vi "VCS Set Operation Mode.vi"(8 "error in (no error)":errorcluster, 10 "modes of operations":i8(ring)=1 items=["Profile Position Mode"=1, "Profile Velocity Mode"=3, "Homing Mode"=6, "Interpolated Position Mode"=7, "Position Mode"=-1, "Velocity Mode"=-2, "Current Mode"=-3, "Master Encoder Mode"=-5, "Step Direction Mode"=-6], 11 "axis in":cluster{"keyHandle":u32, "nodeId":u16}={"keyHandle"=0, "nodeId"=1}) -> (0 "error out":errorcluster, 3 "axis out":cluster{"keyHandle":u32, "nodeId":u16}={"keyHandle"=0, "nodeId"=1})   [LabVIEW 2018]
doc: "<B>VCS Set Operation Mode</B> sets the operation mode."
uses:
  Resources/EposCmd.dll
  Resources/EposCmd64.dll
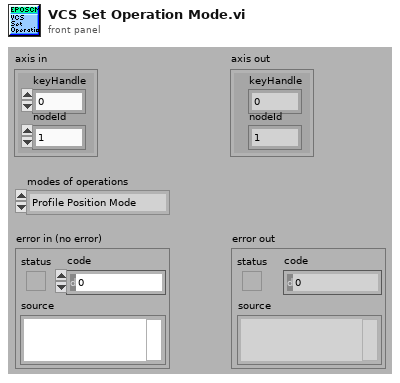
[diagram p1: front panel]
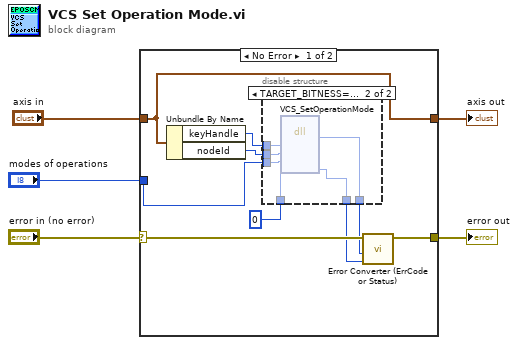
[diagram p0: block diagram]
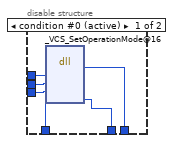
[diagram p2: hidden frame]
diagram:
  n1 = case shown="No Error" "error in (no error)" {
    selector: "error in (no error)" -> [w14 w28]
    tunnel: [w13 w28] -> w4
    tunnel: "modes of operations" -> [w11 _]
    tunnel: "axis in" -> [w8 w27]
    tunnel: [w8 w27] -> w1
    frame No Error {
      n2 = Unbundle By Name(w8) -> ("keyHandle"=w10:u32, "nodeId"=w9:u16)
      n3 = disable-structure shown="TARGET_BITNESS==64" {
        disable-tunnel: [w20 w26] -> w12
        disable-tunnel: w11 -> [w19 w25]
        disable-tunnel: w10 -> [w18 w24]
        disable-tunnel: w9 -> [w17 w23]
        disable-tunnel: u32 0 ("pErrorCode") -> [w16 w22]
        disable-tunnel: [w15 w21] -> w6
        frame condition #0 (active) {
          n4 = dll-call lib="C:/Projeto em LabVIEW/EPOS-LabVIEW-Instrument-Driver-En/LabVIEW/maxon EPOS/Resources/EposCmd.*" fn="_VCS_SetOperationMode@16"("KeyHandle"=w18, "NodeId"=w17, "Mode"=w19, "pErrorCode"=w16) -> (w15:i32, "pErrorCode"=w20:u32)  [unwired: 6 in, 2 out]
        }
        frame condition #1 {
          n5 = dll-call lib="C:/setup/Resources/EposCmd64.*" fn="VCS_SetOperationMode" ("EposCmd.dll:_VCS_SetOperationMode@16")("KeyHandle"=w24, "NodeId"=w23, "Mode"=w25, "pErrorCode"=w22) -> ("Rückgabetyp"=w21:i32, "pErrorCode"=w26:u32)  [unwired: 6 in, 2 out]
        }
      }
      n6 = call "Error Converter (ErrCode or Status).vi"("error code"=w12, "return type"=w6, "error in (no error)"=w14) -> ("error out"=w13:errorcluster)  [unwired: 7 in]
    }
    frame Error {
    }
  }
  "error out" <- w4
  "axis out" <- w1
